vi "JKISM++ Example - Caller is JKISM.vi"() -> ()   [LabVIEW 2014]
uses:
  user.lib/_NEVSTOP/JKI State Machine++/_Polymophic/Build Asynchronous Message with Arguments.vi
  user.lib/_NEVSTOP/JKI State Machine++/_Polymophic/Build No-Reply Asynchronous Message with Arguments.vi
  user.lib/_NEVSTOP/JKI State Machine++/_Polymophic/Build Register Status Message.vi
  user.lib/_NEVSTOP/JKI State Machine++/_Polymophic/Build Unregister Status Message.vi
  user.lib/_NEVSTOP/JKI State Machine++/_Polymophic/Build Synchronous Message with Arguments.vi
  user.lib/_NEVSTOP/JKI State Machine++/_Support/JKISMQ/_Obtain JKISMQ.vi
  user.lib/_NEVSTOP/JKI State Machine++/_Support/FGV-BroadcastRegistry/Cache-Broadcast Registry Search Result.vi
  user.lib/_NEVSTOP/JKI State Machine++/AdvanceAPI/JKISM++ Register Status Change.vi
  user.lib/_NEVSTOP/JKI State Machine++/AdvanceAPI/JKISM++ Unregister Status Change.vi
  user.lib/_NEVSTOP/JKI State Machine++/_Support/JKISMQ/_Create Resp Queue.vi
  user.lib/_NEVSTOP/JKI State Machine++/_Support/JKISMQ/_Unlock JKISMQ.vi
  user.lib/_NEVSTOP/JKI State Machine++/_Support/JKISMQ/_Lock State JKISMQ.vi
  user.lib/_NEVSTOP/JKI State Machine++/_Support/JKISMQ/_Release JKISMQ.vi
  user.lib/_NEVSTOP/JKI State Machine++/AdvanceAPI/JKISM++ Make String Arguments Safe.vi
  user.lib/_NEVSTOP/JKI State Machine++/_Support/Message/Parse State with Arguments String.vi
  user.lib/_NEVSTOP/JKI State Machine++/Utility/Trim Both Whitespace.vi
  user.lib/_NEVSTOP/JKI State Machine++/_Support/JKISMQ/_Input Name to JKISM Mode.vi
  user.lib/_NEVSTOP/JKI State Machine++/Utility/uuid.vi
  user.lib/_NEVSTOP/JKI State Machine++/_Support/KeyWords.vi
  user.lib/_NEVSTOP/JKI State Machine++/_Support/JKISMQ/_JKISMQFGV.vi
  user.lib/_NEVSTOP/JKI State Machine++/_Support/GlobalEvent/FGV-GlobalEventRef.vi
  user.lib/_NEVSTOP/JKI State Machine++/_Support/JKISMQ/_Dequeue JKISMQ.vi
  user.lib/_NEVSTOP/JKI State Machine++/_Support/JKISMQ/_Enqueue JKISMQ.vi
  user.lib/_NEVSTOP/JKI State Machine++/_Support/GlobalEvent/FGV-StatusChangeEventRef.vi
  user.lib/_NEVSTOP/JKI State Machine++/_Support/FGV-BroadcastRegistry/global-Broadcast Cache Change Flag.vi
  user.lib/_NEVSTOP/JKI State Machine++/_Support/FGV-BroadcastRegistry/FGV-BroadcastRegistry.vi
  user.lib/_NEVSTOP/JKI State Machine++/JKI State Machine++.lvlib
panel:
  in  "UI: Front Panel State >> Close":bool
  in  "UI: Front Panel State >> Open":bool
  in  "Level":dbl min=0.0 max=1.0 step=0.1
  in  "Target Module":string(combo)="SubModule0"
  in  "API: Stop":bool
  in  "API: Start":bool
  in  "Unregister All Status Change":bool
  in  "Register All Status Change":bool
  in  "API: Get Level(Async)":bool
  out "State History of Main":string
  # "1. The purpose of this example is to demonstrate how to invoke the JKISM module in the JKISM++ framework program. In this scenario, inter-module communication solely relies on message string queue operations. You can generate a Message string using the \"Build Message with Arguments++.vi\" function. Alternatively, if you are familiar with the rules, you can directly utilize message description strings. \n\nThis example synchronously calls two instances of \"JKISM-Reuse Module.vi\", providing dynamic subscription to status and manipulation of the underlying Module through the API."
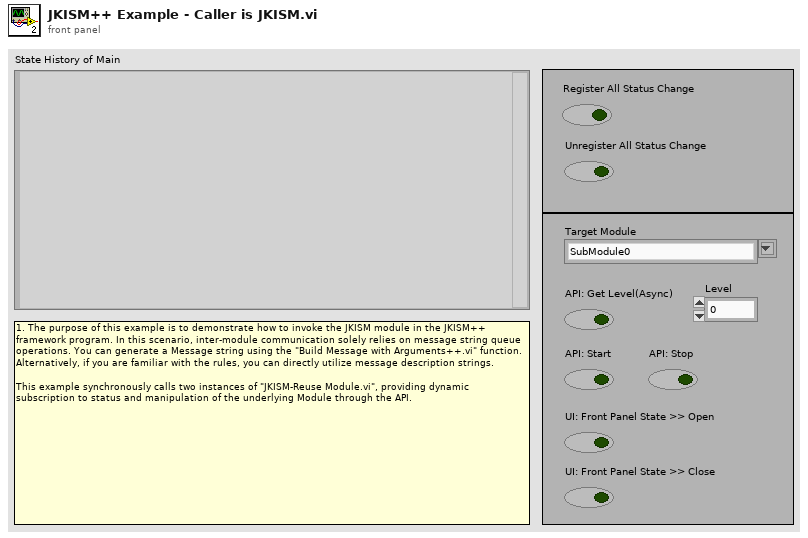
[diagram p1: front panel]
types:
  T1 = enum32{"Invalid", "Standard", "Closed", "Hidden", "Minimized", "Maximized"}
  T2 = enum32{"invalid app kind", "Development System", "Run Time System", "Student Edition", "Embedded LabVIEW", "Evaluation", "Custom"}
  T3 = cluster{"Core":cluster{"Current VI Reference":refnum<vi>, "Close Panel on Exit?":bool}, "Your Boolean data":bool, "Your string data":string, "Active Module":string}
  T4 = cluster{"Current VI Reference":refnum<vi>, "Close Panel on Exit?":bool}
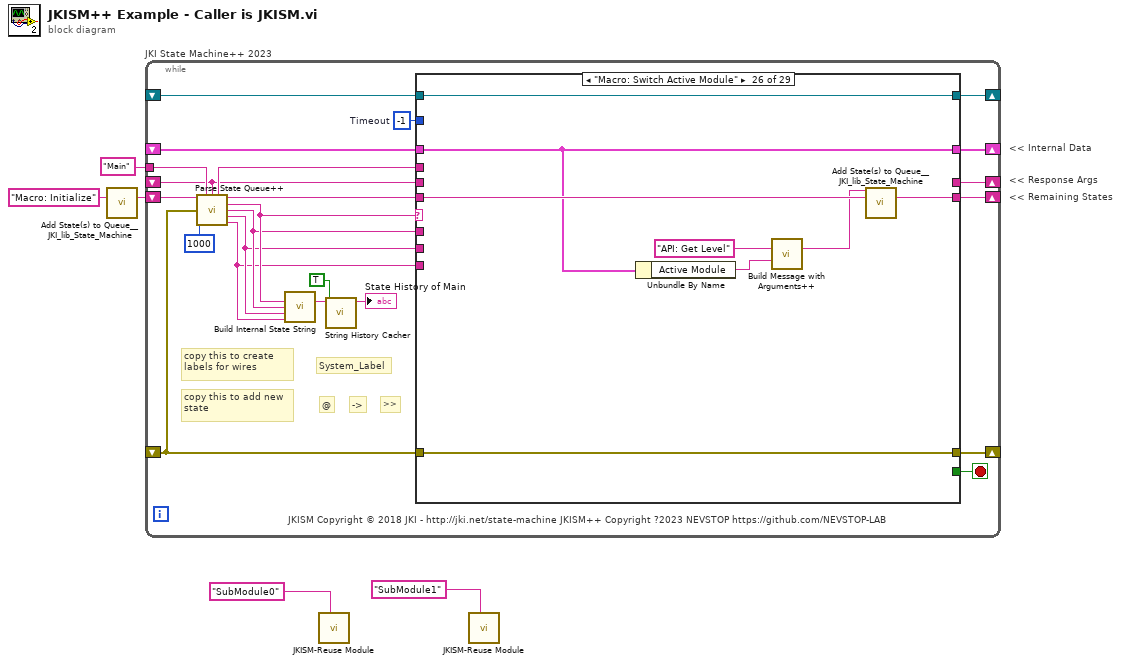
[diagram p0: block diagram]
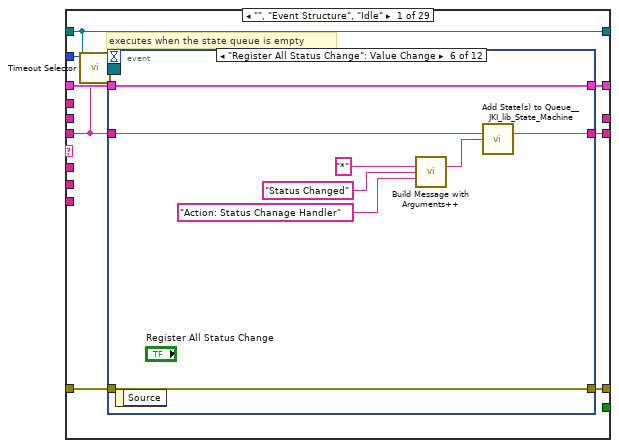
[diagram p2: hidden frame]
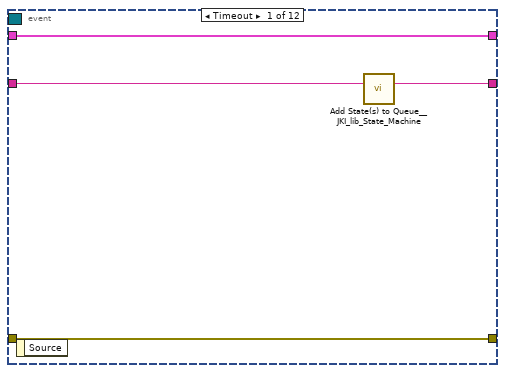
[diagram p3: hidden frame]
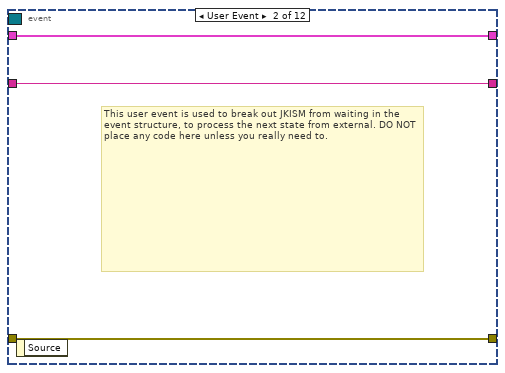
[diagram p4: hidden frame]
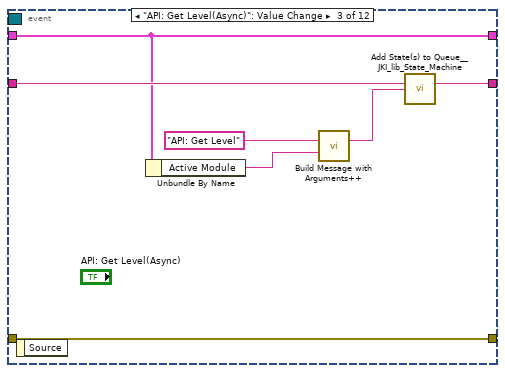
[diagram p5: hidden frame]
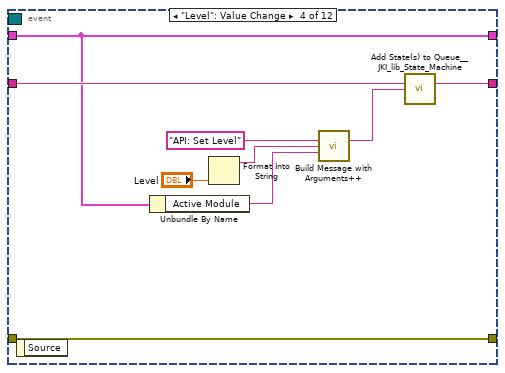
[diagram p6: hidden frame]
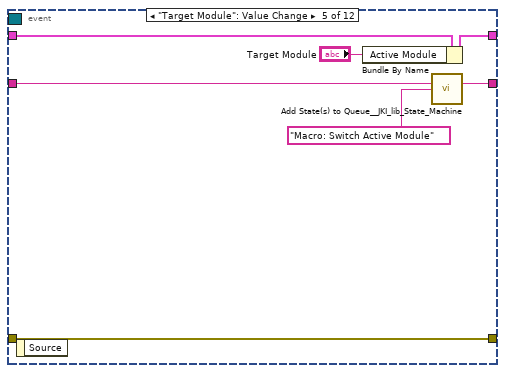
[diagram p7: hidden frame]
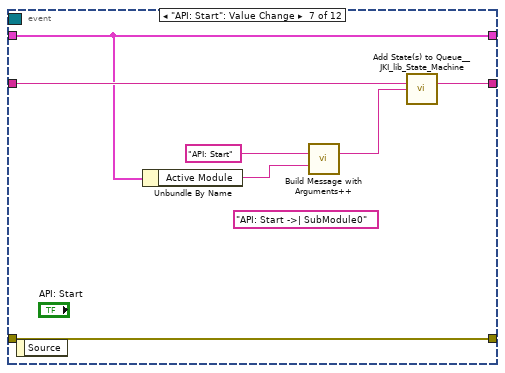
[diagram p8: hidden frame]
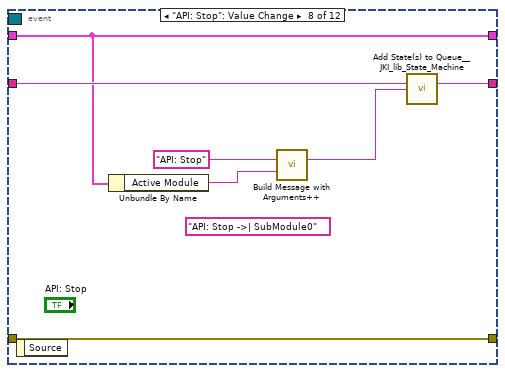
[diagram p9: hidden frame]
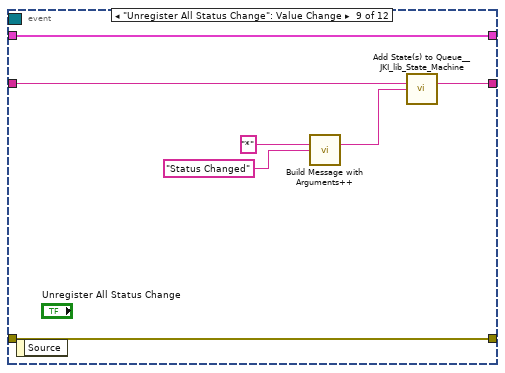
[diagram p10: hidden frame]
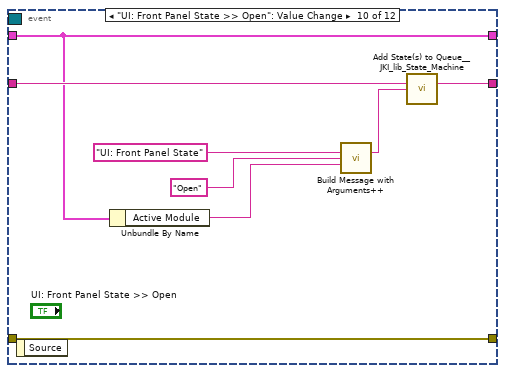
[diagram p11: hidden frame]
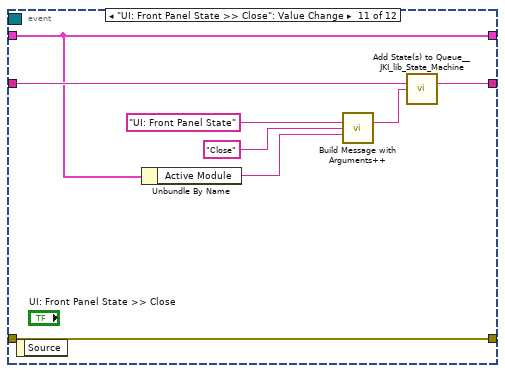
[diagram p12: hidden frame]
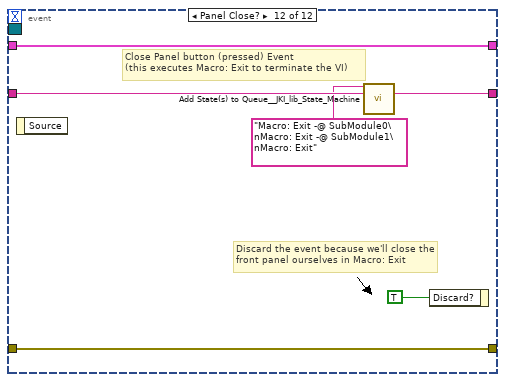
[diagram p13: hidden frame]
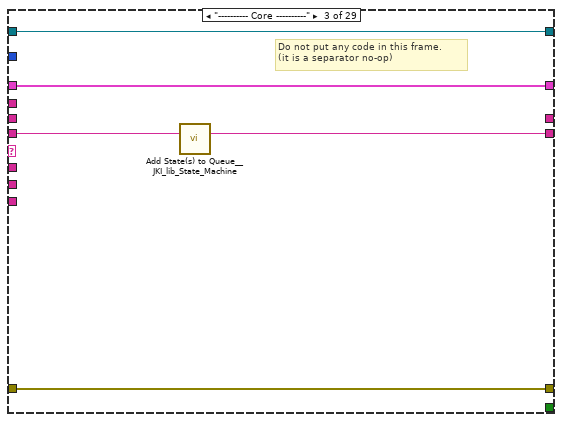
[diagram p15: hidden frame]
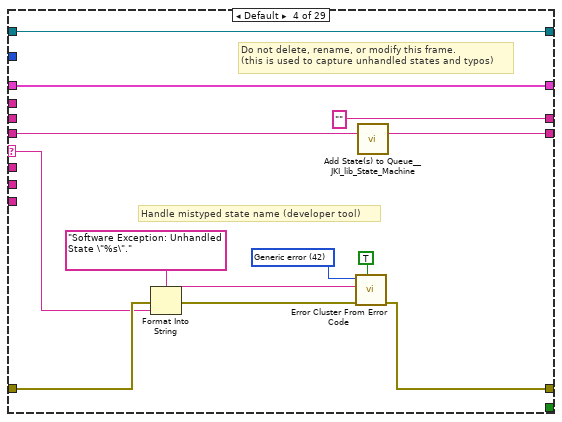
[diagram p16: hidden frame]
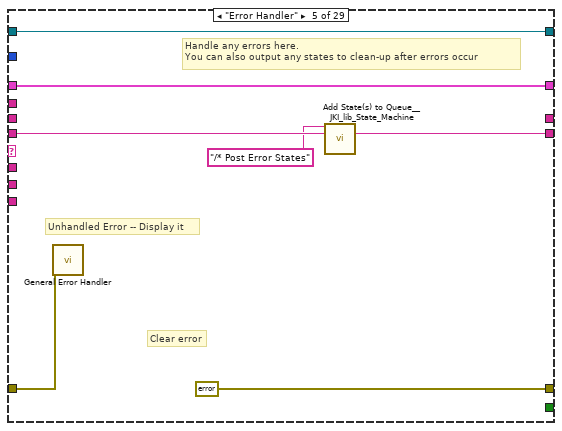
[diagram p17: hidden frame]
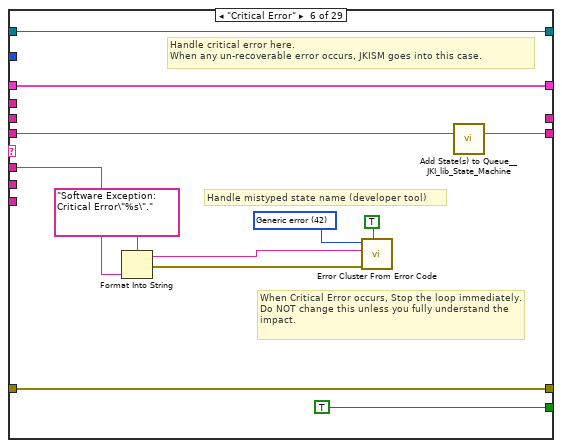
[diagram p18: hidden frame]
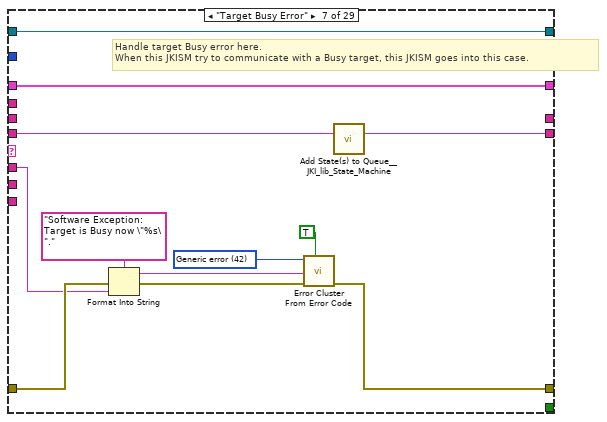
[diagram p19: hidden frame]
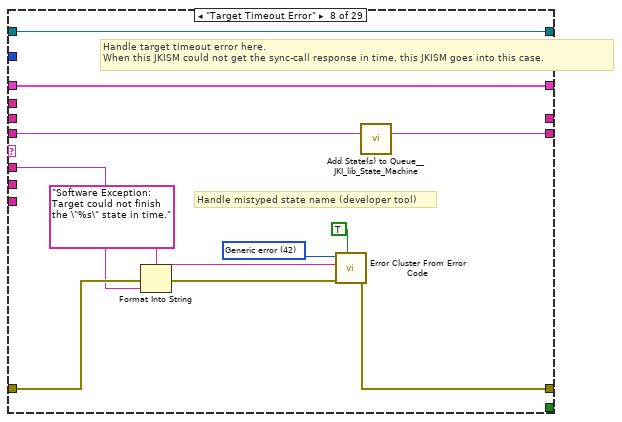
[diagram p20: hidden frame]
diagram:
  # "<< Internal Data"
  # "<< Response Args"
  # "<< Remaining States"
  n1 = call <vilib>:"Add State(s) to Queue__JKI_lib_State_Machine.vi"("State(s) in (\"\")"="Macro: Initialize") -> ("States Out"=w5:string)  [unwired: 14 in]
  n2 = while "JKI State Machine++ 2023" {
    shift-right: [w23] -> _
    shift-left: _ -> [w22]
    shift-right: [w26] -> _
    shift-left: _ -> [w20]
    shift-right: [w25] -> _
    shift-left: w5 -> [w27]
    tunnel: "Main" ("Name(\"\" to use uuid)") -> [w15]
    shift-right: [w18] -> _
    shift-left: _ -> [w7]
    shift-right: [w17] -> _
    shift-left: _ -> [w16]
    stop <- w24 stop-if-true
    w21 = -1  # Timeout
    # "JKISM Copyright © 2018 JKI - http://jki.net/state-machine JKISM++ Copyright ?2023 NEVSTOP https://github.com/NEVSTOP-LAB"
    # "copy this to add new state"
    # ">>"
    # "->"
    # "@"
    # "copy this to create labels for wires"
    # "System_Label"
    n3 = call "Parse State Queue++.vi"("State Queue"=w27, "Name(\"\" to use uuid)"=w15, "Response Arguments"=w7, "Error In (no error)"=w20, "Response Timeout(5000ms)"=1000 ("Response Timeout(1000ms)")) -> ("Name Used"=w8:string, "Remaining States"=w28:string, "Current State"=w12:string, "Arguments"=w11:string, "Argument - State"=w10:string, "From Who"=w9:string)  [unwired: 5 in]
    n4 = call "Build Internal State String.vi"("State"=w12, "Arguments (\"\")"=w11, "Arg-State (\"\")"=w10, "Source (\"\")"=w9) -> ("State with Arguments"=w13:string)  [unwired: 11 in]
    n5 = call "String History Cacher.vi"("Include Timestamp(T)"=TRUE ("Include Timestamp(F)"), "String"=w13) -> ("String Cache"=→"State History of Main":string)  [unwired: 9 in]
    n6 = case shown="\"Macro: Switch Active Module\"" w12 {
      selector: w12 -> [_ _ _ w130 _ _ _ _ _ _ _ _ _ _ _ _ _ _ _ _ _ _ _ _ _ _ _ _ _]
      tunnel: w28 -> [w29 w121 w127 w134 w147 w157 w160 w177 w189 w200 w206 w221 w227 w232 w241 w248 w253 w259 w263 w269 w275 w282 w294 w364 w370 w375 w389 w392 w396]
      tunnel: w11 -> [_ _ _ _ _ w150 w162 w173 w185 w196 _ _ _ _ _ _ _ _ _ _ _ w277 w288 _ _ _ _ _ _]
      tunnel: w22 -> [w36 w120 w124 w132 w144 w158 w164 w175 w187 w199 w205 w214 w225 w229 _ w243 w250 w258 w262 w266 w271 w280 w290 w361 w367 w373 w386 w391 w395]
      tunnel: [w35 w122 w125 w136 errorcluster {"status"=FALSE, "code"=0, "source"=""} ("error out") w159 w167 w179 w191 w201 w207 w218 w224 w230 w238 w244 w251 w254 w261 w267 w273 w278 w291 w362 w368 w378 w387 w393 w397] -> w26
      tunnel: w20 -> [w34 w122 w125 w135 w143 w159 w166 w178 w190 w201 w207 w218 w224 w230 w238 w245 w251 _ w264 w267 w273 w279 w292 w362 w368 w378 w387 w393 w397]
      tunnel: [w37 w121 w126 w133 w146 w156 w165 w176 w188 w200 w206 w220 w226 w231 w240 w247 w252 w259 w263 w268 w274 w281 w293 w363 w369 w376 w388 w392 w396] -> w25
      tunnel: [_ _ _ _ _ TRUE _ _ _ _ _ _ TRUE _ _ _ _ _ _ _ _ _ _ _ _ _ _ _ _] -> w24
      tunnel: [w33 w120 w124 w132 w144 w158 w164 w175 w187 w199 w205 w219 w225 w229 w239 w243 w250 w258 w262 w266 w271 w280 w290 w361 w367 w373 w386 w391 w395] -> w23
      tunnel: w21 -> [w32 _ _ _ _ _ _ _ _ _ _ _ _ _ _ _ _ _ _ _ _ _ _ _ _ _ _ _ _]
      tunnel: w9 -> [_ _ _ _ _ _ _ _ _ _ _ _ _ _ _ _ _ _ _ _ _ _ _ _ _ _ _ _ _]
      tunnel: w10 -> [_ _ _ _ _ _ _ _ _ w197 _ _ _ _ _ _ _ _ _ _ _ _ _ _ _ _ _ _ _]
      tunnel: [_ _ _ "" _ _ _ _ _ _ _ _ _ _ _ _ _ _ _ _ _ _ _ _ _ _ _ _ _] -> w18
      tunnel: [w31 w119 w123 w128 w141 w148 w161 w172 w184 w198 w204 w208 w222 w228 w234 w242 w249 w257 w260 w265 w272 w276 w287 w360 w365 w377 w379 w390 w394] -> w17
      tunnel: w16 -> [w31 w119 w123 w128 w141 w148 w161 w172 w184 w198 w204 w208 w222 w228 w234 w242 w249 _ w260 w265 w272 w276 w287 w360 w365 w377 w379 w390 w394]
      tunnel: w8 -> [_ _ _ _ _ _ _ _ _ _ _ _ _ _ _ _ _ w256 _ _ _ _ _ _ _ _ _ _ _]
      tunnel: w7 -> [_ _ _ _ _ _ _ _ _ _ _ _ _ _ _ _ _ _ _ _ _ _ _ _ _ _ _ _ _]
      frame "", "Event Structure", "Idle" {
        # "executes when the state queue is empty"
        n7 = call "Timeout Selector.vi"("Remaining States"=w29, "Timeout Expected"=w32) -> ("Timeout"=w30:i32)  [unwired: 5 in]
        n8 = event shown="[5] \"Register All Status Change\": Value Change" {
          selector: w31 -> [_ _ _ _ _ _ _ _ _ _ _ _]
          dyn-events: _ -> [_ _ _ _ _ _ _ _ _ _ _ _]
          timeout: w30 -> [_ _ _ _ _ _ _ _ _ _ _ _]
          tunnel: w29 -> [w41 w43 w50 w59 w64 w73 w81 w88 w94 w103 w111 w118]
          tunnel: [w40 w43 w49 w58 w65 w72 w80 w87 w93 w102 w110 w117] -> w37
          tunnel: w36 -> [w38 w44 w46 w53 w66 w74 w77 w84 w95 w101 w108 w115]
          tunnel: [w39 w42 w51 w60 w67 w75 w82 w89 w96 w104 w112 w116] -> w35
          tunnel: w34 -> [w39 w42 w51 w60 w67 w75 w82 w89 w96 w104 w112 w116]
          tunnel: [w38 w44 w46 w53 w62 w74 w77 w84 w95 w101 w108 w115] -> w33
          event Timeout {
            n9 = event-data() -> ()  [unwired: 1 in, 1 out]
            n10 = call <vilib>:"Add State(s) to Queue__JKI_lib_State_Machine.vi"("State(s) in (\"\")"=w41) -> ("States Out"=w40:string)  [unwired: 14 in]
          }
          event User Event {
            # "This user event is used to break out JKISM from waiting in the event structure, to process the next state from external. DO NOT place any code here unless you really need to."
            n11 = event-data() -> ()  [unwired: 1 in, 1 out]
          }
          event "API: Get Level(Async)": Value Change {
            n12 = event-data() -> ()  [unwired: 1 in, 1 out]
            n13 = Unbundle By Name(w46) -> ("Active Module"=w45:string)
            n14 = call-poly "Build Message with Arguments++.vi"("State with Arguments"="API: Get Level" ("State(s) in Front (\"\")"), "Target Module (\"\")"=w45) -> ("State with Arguments"=w47:string)  [unwired: 13 in]
            n15 = call <vilib>:"Add State(s) to Queue__JKI_lib_State_Machine.vi"("State(s) in (\"\")"=w50, "State(s) at Back (\"\")"=w47) -> ("States Out"=w49:string)  [unwired: 13 in]
          }
          event "Level": Value Change {
            n16 = event-data() -> ()  [unwired: 1 in, 1 out]
            n17 = Unbundle By Name(w53) -> ("Active Module"=w52:string)
            n18 = Format Into String("Level") -> (resulting string=w54:string)  [unwired: 3 in, 1 out]
            n19 = call-poly "Build Message with Arguments++.vi"("State with Arguments"="API: Set Level" ("State(s) in Front (\"\")"), "Arguments (\"\")"=w54, "Target Module (\"\")"=w52) -> ("State with Arguments"=w56:string)  [unwired: 12 in]
            n20 = call <vilib>:"Add State(s) to Queue__JKI_lib_State_Machine.vi"("State(s) in (\"\")"=w59, "State(s) at Back (\"\")"=w56) -> ("States Out"=w58:string)  [unwired: 13 in]
          }
          event "Target Module": Value Change {
            n21 = event-data() -> ()  [unwired: 1 in, 1 out]
            n22 = Bundle By Name(cluster=w66, "Active Module"="Target Module") -> (w62:T3)
            n23 = call <vilib>:"Add State(s) to Queue__JKI_lib_State_Machine.vi"("State(s) in (\"\")"=w64, "State(s) at Back (\"\")"="Macro: Switch Active Module" ("State(s) at Back (\"\")")) -> ("States Out"=w65:string)  [unwired: 13 in]
          }
          event "Register All Status Change": Value Change {
            n24 = event-data() -> ()  [unwired: 1 in, 1 out]
            n25 = call-poly "Build Message with Arguments++.vi"("Source JKISM Name (* as Default)"="*", "Status"="Status Changed", "Response Message (if \"\", same as Source Message)"="Action: Status Chanage Handler" ("Status")) -> ("State with Arguments"=w68:string)  [unwired: 12 in]
            n26 = call <vilib>:"Add State(s) to Queue__JKI_lib_State_Machine.vi"("State(s) in (\"\")"=w73, "State(s) at Back (\"\")"=w68) -> ("States Out"=w72:string)  [unwired: 13 in]
          }
          event "API: Start": Value Change {
            (unwired) "API: Start ->| SubModule0" ("State(s) in Front (\"\")")
            n27 = event-data() -> ()  [unwired: 1 in, 1 out]
            n28 = Unbundle By Name(w77) -> ("Active Module"=w76:string)
            n29 = call-poly "Build Message with Arguments++.vi"("State with Arguments"="API: Start" ("State(s) in Front (\"\")"), "Target Module (\"\")"=w76) -> ("State with Arguments"=w78:string)  [unwired: 13 in]
            n30 = call <vilib>:"Add State(s) to Queue__JKI_lib_State_Machine.vi"("State(s) in (\"\")"=w81, "State(s) at Back (\"\")"=w78) -> ("States Out"=w80:string)  [unwired: 13 in]
          }
          event "API: Stop": Value Change {
            (unwired) "API: Stop ->| SubModule0" ("State(s) in Front (\"\")")
            n31 = event-data() -> ()  [unwired: 1 in, 1 out]
            n32 = Unbundle By Name(w84) -> ("Active Module"=w83:string)
            n33 = call-poly "Build Message with Arguments++.vi"("State with Arguments"="API: Stop" ("State(s) in Front (\"\")"), "Target Module (\"\")"=w83) -> ("State with Arguments"=w85:string)  [unwired: 13 in]
            n34 = call <vilib>:"Add State(s) to Queue__JKI_lib_State_Machine.vi"("State(s) in (\"\")"=w88, "State(s) at Back (\"\")"=w85) -> ("States Out"=w87:string)  [unwired: 13 in]
          }
          event "Unregister All Status Change": Value Change {
            n35 = event-data() -> ()  [unwired: 1 in, 1 out]
            n36 = call-poly "Build Message with Arguments++.vi"("Source JKISM Name (* as Default)"="*", "Status"="Status Changed") -> ("State with Arguments"=w90:string)  [unwired: 13 in]
            n37 = call <vilib>:"Add State(s) to Queue__JKI_lib_State_Machine.vi"("State(s) in (\"\")"=w94, "State(s) at Back (\"\")"=w90) -> ("States Out"=w93:string)  [unwired: 13 in]
          }
          event "UI: Front Panel State >> Open": Value Change {
            n38 = event-data() -> ()  [unwired: 1 in, 1 out]
            n39 = Unbundle By Name(w101) -> ("Active Module"=w100:string)
            n40 = call-poly "Build Message with Arguments++.vi"("State with Arguments"="UI: Front Panel State" ("JKISM Name"), "Arguments (\"\")"="Open" ("JKISM Name"), "Target Module (\"\")"=w100) -> ("State with Arguments"=w99:string)  [unwired: 12 in]
            n41 = call <vilib>:"Add State(s) to Queue__JKI_lib_State_Machine.vi"("State(s) in (\"\")"=w103, "State(s) at Back (\"\")"=w99) -> ("States Out"=w102:string)  [unwired: 13 in]
          }
          event "UI: Front Panel State >> Close": Value Change {
            n42 = event-data() -> ()  [unwired: 1 in, 1 out]
            n43 = Unbundle By Name(w108) -> ("Active Module"=w107:string)
            n44 = call-poly "Build Message with Arguments++.vi"("State with Arguments"="UI: Front Panel State" ("JKISM Name"), "Arguments (\"\")"="Close" ("JKISM Name"), "Target Module (\"\")"=w107) -> ("State with Arguments"=w106:string)  [unwired: 12 in]
            n45 = call <vilib>:"Add State(s) to Queue__JKI_lib_State_Machine.vi"("State(s) in (\"\")"=w111, "State(s) at Back (\"\")"=w106) -> ("States Out"=w110:string)  [unwired: 13 in]
          }
          event Panel Close? {
            # "Discard the event because we'll close the front panel ourselves in Macro: Exit"
            # "Close Panel button (pressed) Event\n(this executes Macro: Exit to terminate the VI)"
            n46 = event-data() -> ()  [unwired: 1 in, 1 out]
            n47 = call <vilib>:"Add State(s) to Queue__JKI_lib_State_Machine.vi"("State(s) in Front (\"\")"="Macro: Exit -@ SubModule0\nMacro: Exit -@ SubModule1\nMacro: Exit", "State(s) in (\"\")"=w118) -> ("States Out"=w117:string)  [unwired: 13 in]
            n48 = event-data("Discard?"=TRUE) -> ()  [unwired: 1 in, 1 out]
          }
        }
      }
      frame "JKISM++ Documentation" {
        # "Commenting:\nTo add a comment use \"//\" or \"#\" and all text to the right will be ignored\nCommenting Example:\nUI: Initialize // This initializes the UI\n# This whole line is a comment\n// Another comment line"
        # "State Syntax:\nStateCategory: State >> Argument @ JKISMName\nStateCategory: State >> Argument -> JKISMName\n\nLine Terminator: Line feed"
        # "JKISM++ Documentation"
      }
      frame "---------- Core ----------" {
        # "Do not put any code in this frame.\n(it is a separator no-op)"
        n49 = call <vilib>:"Add State(s) to Queue__JKI_lib_State_Machine.vi"("State(s) in (\"\")"=w127) -> ("States Out"=w126:string)  [unwired: 14 in]
      }
      frame Default {
        w139 = 42 items=["No error", "Argument error", "Memory is full", "Out of zone", "End of file", "File already open", "Generic file I/O error", "File not found", "File permission error", "Disk is full", "Duplicate path", "Too many files open", "System feature not enabled", "Resource file not found", "Cannot add resource", "Resource not found", "Image not found", "Image memory error", "Pen does not exist", "Config type invalid", "Config token not found", "Config parse error", "Config memory error", "Bad external code format", "Bad external code offset", "External code not present", "Null window", "Destroy window error", "Null menu", "Print aborted", "Bad print record", "Print driver error", "Windows error during printing", "Memory error during printing", "Print dialog error", "Generic print error", "Invalid device refnum", "Device not found", "Device parameter error", "Device unit error", "Cannot open device", "Device call aborted", "Generic error", "Cancelled by user", "Object ID too low", "Object ID too high", "Object not in heap", "Unknown heap", "Unknown object (invalid DefProc)", "Unknown object (DefProc not in table)", "Message out of range", "Invalid (null) method", "Unknown message", "Manager call not supported", "Bad address", "Network operation in progress", "Network operation timed out", "Connection is busy", "Network attribute not supported", "Network error", "Address in use", "System out of memory", "Connection aborted", "Connection refused", "Not connected", "Already connected", "Connection closed", "Initialization error (interapplication manager)", "Bad occurrence", "Wait on unbound occurrence handler", "Occurrence queue overflow", "Datalog type conflict", "Unused", "Unrecognized type (interapplication manager)", "Memory corrupt", "Failed to make temporary DLL", "Old CIN version", "Drag socket not found", "Failed to load drop-object", "Failed to register OLE object", "Failed to release OLE object", "Format specifier type mismatch", "Unknown format specifier", "Too few format specifiers", "Too many format specifiers", "Scan failed", "Newer CIN version", "Error converting to variant", "Runtime menu error", "Password tampered", "Variant attribute not found", "Incompatible variant data type", "Event data is not available", "Event Store is not present", "Occurrence is not found", "Event Queue is not created", "Event info is not available", "Refnum passed is NULL", "Error retrieving Class GUID", "Error retrieving CoClass GUID", "Error retrieving TypeLib GUID.", "Bad built application magic bytes.", "Specific driver is different from the specific driver associated with the Logical Name.", "There is no session opened to the class driver.", "Max Error", "MAX - Error with config objects", "MAX - Error loading configuration", "MAX - Group not supported"]
        # "Do not delete, rename, or modify this frame.\n(this is used to capture unhandled states and typos)"
        # "Handle mistyped state name (developer tool)"
        n50 = Format Into String(format string="Software Exception: Unhandled State \"%s\"." ("message"), error in=w135, w130) -> (resulting string=w138:string, error out=w137:errorcluster)  [unwired: 1 in]
        n51 = call <vilib>:"Error Cluster From Error Code.vi"("show call chain? (False)"=TRUE, "error in (no error)"=w137, "error message (\"\")"=w138, "error code (0)"=w139) -> ("error out"=w136:errorcluster)  [unwired: 5 in]
        n52 = call <vilib>:"Add State(s) to Queue__JKI_lib_State_Machine.vi"("State(s) in (\"\")"=w134) -> ("States Out"=w133:string)  [unwired: 14 in]
      }
      frame "Error Handler" {
        # "Unhandled Error -- Display it"
        # "Handle any errors here.\nYou can also output any states to clean-up after errors occur"
        # "Clear error"
        n53 = call <vilib>:"General Error Handler.vi"("error in (no error)"=w143) -> ()  [unwired: 10 in, 5 out]
        n54 = call <vilib>:"Add State(s) to Queue__JKI_lib_State_Machine.vi"("State(s) in Front (\"\")"="/* Post Error States", "State(s) in (\"\")"=w147) -> ("States Out"=w146:string)  [unwired: 13 in]
      }
      frame "Critical Error" {
        w154 = 42 items=["No error", "Argument error", "Memory is full", "Out of zone", "End of file", "File already open", "Generic file I/O error", "File not found", "File permission error", "Disk is full", "Duplicate path", "Too many files open", "System feature not enabled", "Resource file not found", "Cannot add resource", "Resource not found", "Image not found", "Image memory error", "Pen does not exist", "Config type invalid", "Config token not found", "Config parse error", "Config memory error", "Bad external code format", "Bad external code offset", "External code not present", "Null window", "Destroy window error", "Null menu", "Print aborted", "Bad print record", "Print driver error", "Windows error during printing", "Memory error during printing", "Print dialog error", "Generic print error", "Invalid device refnum", "Device not found", "Device parameter error", "Device unit error", "Cannot open device", "Device call aborted", "Generic error", "Cancelled by user", "Object ID too low", "Object ID too high", "Object not in heap", "Unknown heap", "Unknown object (invalid DefProc)", "Unknown object (DefProc not in table)", "Message out of range", "Invalid (null) method", "Unknown message", "Manager call not supported", "Bad address", "Network operation in progress", "Network operation timed out", "Connection is busy", "Network attribute not supported", "Network error", "Address in use", "System out of memory", "Connection aborted", "Connection refused", "Not connected", "Already connected", "Connection closed", "Initialization error (interapplication manager)", "Bad occurrence", "Wait on unbound occurrence handler", "Occurrence queue overflow", "Datalog type conflict", "Unused", "Unrecognized type (interapplication manager)", "Memory corrupt", "Failed to make temporary DLL", "Old CIN version", "Drag socket not found", "Failed to load drop-object", "Failed to register OLE object", "Failed to release OLE object", "Format specifier type mismatch", "Unknown format specifier", "Too few format specifiers", "Too many format specifiers", "Scan failed", "Newer CIN version", "Error converting to variant", "Runtime menu error", "Password tampered", "Variant attribute not found", "Incompatible variant data type", "Event data is not available", "Event Store is not present", "Occurrence is not found", "Event Queue is not created", "Event info is not available", "Refnum passed is NULL", "Error retrieving Class GUID", "Error retrieving CoClass GUID", "Error retrieving TypeLib GUID.", "Bad built application magic bytes.", "Specific driver is different from the specific driver associated with the Logical Name.", "There is no session opened to the class driver.", "Max Error", "MAX - Error with config objects", "MAX - Error loading configuration", "MAX - Group not supported"]
        # "Handle critical error here.\nWhen any un-recoverable error occurs, JKISM goes into this case."
        # "When Critical Error occurs, Stop the loop immediately. Do NOT change this unless you fully understand the impact."
        # "Handle mistyped state name (developer tool)"
        n55 = Format Into String(format string="Software Exception: Critical Error\"%s\"." ("message"), w150) -> (resulting string=w153:string, error out=w152:errorcluster)  [unwired: 2 in]
        n56 = call <vilib>:"Error Cluster From Error Code.vi"("show call chain? (False)"=TRUE, "error in (no error)"=w152, "error message (\"\")"=w153, "error code (0)"=w154) -> ()  [unwired: 5 in, 1 out]
        n57 = call <vilib>:"Add State(s) to Queue__JKI_lib_State_Machine.vi"("State(s) in (\"\")"=w157) -> ("States Out"=w156:string)  [unwired: 14 in]
      }
      frame "Target Busy Error" {
        w170 = 42 items=["No error", "Argument error", "Memory is full", "Out of zone", "End of file", "File already open", "Generic file I/O error", "File not found", "File permission error", "Disk is full", "Duplicate path", "Too many files open", "System feature not enabled", "Resource file not found", "Cannot add resource", "Resource not found", "Image not found", "Image memory error", "Pen does not exist", "Config type invalid", "Config token not found", "Config parse error", "Config memory error", "Bad external code format", "Bad external code offset", "External code not present", "Null window", "Destroy window error", "Null menu", "Print aborted", "Bad print record", "Print driver error", "Windows error during printing", "Memory error during printing", "Print dialog error", "Generic print error", "Invalid device refnum", "Device not found", "Device parameter error", "Device unit error", "Cannot open device", "Device call aborted", "Generic error", "Cancelled by user", "Object ID too low", "Object ID too high", "Object not in heap", "Unknown heap", "Unknown object (invalid DefProc)", "Unknown object (DefProc not in table)", "Message out of range", "Invalid (null) method", "Unknown message", "Manager call not supported", "Bad address", "Network operation in progress", "Network operation timed out", "Connection is busy", "Network attribute not supported", "Network error", "Address in use", "System out of memory", "Connection aborted", "Connection refused", "Not connected", "Already connected", "Connection closed", "Initialization error (interapplication manager)", "Bad occurrence", "Wait on unbound occurrence handler", "Occurrence queue overflow", "Datalog type conflict", "Unused", "Unrecognized type (interapplication manager)", "Memory corrupt", "Failed to make temporary DLL", "Old CIN version", "Drag socket not found", "Failed to load drop-object", "Failed to register OLE object", "Failed to release OLE object", "Format specifier type mismatch", "Unknown format specifier", "Too few format specifiers", "Too many format specifiers", "Scan failed", "Newer CIN version", "Error converting to variant", "Runtime menu error", "Password tampered", "Variant attribute not found", "Incompatible variant data type", "Event data is not available", "Event Store is not present", "Occurrence is not found", "Event Queue is not created", "Event info is not available", "Refnum passed is NULL", "Error retrieving Class GUID", "Error retrieving CoClass GUID", "Error retrieving TypeLib GUID.", "Bad built application magic bytes.", "Specific driver is different from the specific driver associated with the Logical Name.", "There is no session opened to the class driver.", "Max Error", "MAX - Error with config objects", "MAX - Error loading configuration", "MAX - Group not supported"]
        # "Handle target Busy error here.\nWhen this JKISM try to communicate with a Busy target, this JKISM goes into this case."
        n58 = Format Into String(format string="Software Exception: Target is Busy now \"%s\"." ("message"), error in=w166, w162) -> (resulting string=w169:string, error out=w168:errorcluster)  [unwired: 1 in]
        n59 = call <vilib>:"Error Cluster From Error Code.vi"("show call chain? (False)"=TRUE, "error in (no error)"=w168, "error message (\"\")"=w169, "error code (0)"=w170) -> ("error out"=w167:errorcluster)  [unwired: 5 in]
        n60 = call <vilib>:"Add State(s) to Queue__JKI_lib_State_Machine.vi"("State(s) in (\"\")"=w160) -> ("States Out"=w165:string)  [unwired: 14 in]
      }
      frame "Target Timeout Error" {
        w182 = 42 items=["No error", "Argument error", "Memory is full", "Out of zone", "End of file", "File already open", "Generic file I/O error", "File not found", "File permission error", "Disk is full", "Duplicate path", "Too many files open", "System feature not enabled", "Resource file not found", "Cannot add resource", "Resource not found", "Image not found", "Image memory error", "Pen does not exist", "Config type invalid", "Config token not found", "Config parse error", "Config memory error", "Bad external code format", "Bad external code offset", "External code not present", "Null window", "Destroy window error", "Null menu", "Print aborted", "Bad print record", "Print driver error", "Windows error during printing", "Memory error during printing", "Print dialog error", "Generic print error", "Invalid device refnum", "Device not found", "Device parameter error", "Device unit error", "Cannot open device", "Device call aborted", "Generic error", "Cancelled by user", "Object ID too low", "Object ID too high", "Object not in heap", "Unknown heap", "Unknown object (invalid DefProc)", "Unknown object (DefProc not in table)", "Message out of range", "Invalid (null) method", "Unknown message", "Manager call not supported", "Bad address", "Network operation in progress", "Network operation timed out", "Connection is busy", "Network attribute not supported", "Network error", "Address in use", "System out of memory", "Connection aborted", "Connection refused", "Not connected", "Already connected", "Connection closed", "Initialization error (interapplication manager)", "Bad occurrence", "Wait on unbound occurrence handler", "Occurrence queue overflow", "Datalog type conflict", "Unused", "Unrecognized type (interapplication manager)", "Memory corrupt", "Failed to make temporary DLL", "Old CIN version", "Drag socket not found", "Failed to load drop-object", "Failed to register OLE object", "Failed to release OLE object", "Format specifier type mismatch", "Unknown format specifier", "Too few format specifiers", "Too many format specifiers", "Scan failed", "Newer CIN version", "Error converting to variant", "Runtime menu error", "Password tampered", "Variant attribute not found", "Incompatible variant data type", "Event data is not available", "Event Store is not present", "Occurrence is not found", "Event Queue is not created", "Event info is not available", "Refnum passed is NULL", "Error retrieving Class GUID", "Error retrieving CoClass GUID", "Error retrieving TypeLib GUID.", "Bad built application magic bytes.", "Specific driver is different from the specific driver associated with the Logical Name.", "There is no session opened to the class driver.", "Max Error", "MAX - Error with config objects", "MAX - Error loading configuration", "MAX - Group not supported"]
        # "Handle target timeout error here.\nWhen this JKISM could not get the sync-call response in time, this JKISM goes into this case."
        # "Handle mistyped state name (developer tool)"
        n61 = Format Into String(format string="Software Exception: Target could not finish the \"%s\" state in time." ("message"), error in=w178, w173) -> (resulting string=w181:string, error out=w180:errorcluster)  [unwired: 1 in]
        n62 = call <vilib>:"Error Cluster From Error Code.vi"("show call chain? (False)"=TRUE, "error in (no error)"=w180, "error message (\"\")"=w181, "error code (0)"=w182) -> ("error out"=w179:errorcluster)  [unwired: 5 in]
        n63 = call <vilib>:"Add State(s) to Queue__JKI_lib_State_Machine.vi"("State(s) in (\"\")"=w177) -> ("States Out"=w176:string)  [unwired: 14 in]
      }
      frame "Target Error" {
        w194 = 42 items=["No error", "Argument error", "Memory is full", "Out of zone", "End of file", "File already open", "Generic file I/O error", "File not found", "File permission error", "Disk is full", "Duplicate path", "Too many files open", "System feature not enabled", "Resource file not found", "Cannot add resource", "Resource not found", "Image not found", "Image memory error", "Pen does not exist", "Config type invalid", "Config token not found", "Config parse error", "Config memory error", "Bad external code format", "Bad external code offset", "External code not present", "Null window", "Destroy window error", "Null menu", "Print aborted", "Bad print record", "Print driver error", "Windows error during printing", "Memory error during printing", "Print dialog error", "Generic print error", "Invalid device refnum", "Device not found", "Device parameter error", "Device unit error", "Cannot open device", "Device call aborted", "Generic error", "Cancelled by user", "Object ID too low", "Object ID too high", "Object not in heap", "Unknown heap", "Unknown object (invalid DefProc)", "Unknown object (DefProc not in table)", "Message out of range", "Invalid (null) method", "Unknown message", "Manager call not supported", "Bad address", "Network operation in progress", "Network operation timed out", "Connection is busy", "Network attribute not supported", "Network error", "Address in use", "System out of memory", "Connection aborted", "Connection refused", "Not connected", "Already connected", "Connection closed", "Initialization error (interapplication manager)", "Bad occurrence", "Wait on unbound occurrence handler", "Occurrence queue overflow", "Datalog type conflict", "Unused", "Unrecognized type (interapplication manager)", "Memory corrupt", "Failed to make temporary DLL", "Old CIN version", "Drag socket not found", "Failed to load drop-object", "Failed to register OLE object", "Failed to release OLE object", "Format specifier type mismatch", "Unknown format specifier", "Too few format specifiers", "Too many format specifiers", "Scan failed", "Newer CIN version", "Error converting to variant", "Runtime menu error", "Password tampered", "Variant attribute not found", "Incompatible variant data type", "Event data is not available", "Event Store is not present", "Occurrence is not found", "Event Queue is not created", "Event info is not available", "Refnum passed is NULL", "Error retrieving Class GUID", "Error retrieving CoClass GUID", "Error retrieving TypeLib GUID.", "Bad built application magic bytes.", "Specific driver is different from the specific driver associated with the Logical Name.", "There is no session opened to the class driver.", "Max Error", "MAX - Error with config objects", "MAX - Error loading configuration", "MAX - Group not supported"]
        # "Handle target error here.\nWhen this JKISM try to communicate with an un-existed JKISM, this JKISM goes into this case."
        # "Handle mistyped state name (developer tool)"
        n64 = Format Into String(format string="Software Exception: Target \"%s\" does not exists." ("message"), error in=w190, w185) -> (resulting string=w193:string, error out=w192:errorcluster)  [unwired: 1 in]
        n65 = call <vilib>:"Add State(s) to Queue__JKI_lib_State_Machine.vi"("State(s) in (\"\")"=w189) -> ("States Out"=w188:string)  [unwired: 14 in]
        n66 = call <vilib>:"Error Cluster From Error Code.vi"("show call chain? (False)"=TRUE, "error in (no error)"=w192, "error message (\"\")"=w193, "error code (0)"=w194) -> ("error out"=w191:errorcluster)  [unwired: 5 in]
      }
      frame "Async Response", "Response" {
        # "Handle Async-call Response (\"Async Response\" for ->)"
        # "Handle Sync-call Response (\"Response\" for @)"
        n67 = case shown="\"API: Get Level\"" w197 {
          tunnel: w196 -> [_ w203]
          frame "False", Default {
          }
          frame "API: Get Level" {
            n68 = Fract/Exp String To Number(string=w203) -> (number=w202:dbl)  [unwired: 3 in, 1 out]
            n69 = local write "Level"(w202) -> ()
          }
        }
      }
      frame "Async Message Posted" {
        # "Handle post action for async message (->)."
        # "After Async Message is posted (->), JKISM+ goes to this state for post-action. You can use Argument - State to tell which Async Message is called."
      }
      frame "Initialize Core Data" {
        # "Do not delete, rename, or modify this frame.\n(this is used to determine panel behavior on exit)"
        # "originally closed?"
        # "exe?"
        # "If panel starts closed or is an EXE, then close it when we exit"
        n70 = property class="VI"() -> ("FP.State"=w211:T1)  [unwired: 2 in, 2 out]
        n71 = property class="App"() -> ("App.Kind"=w217:T2)  [unwired: 2 in, 2 out]
        n72 = control-ref of="Current VI Reference"() -> (w212:refnum<vi>)
        n73 = Equal?(x=w211, y=T1."Closed" ("Front Panel Window:State")) -> (x = y?=w209:bool)
        n74 = Equal?(x=w217, y=T2."Run Time System" ("Application:Kind")) -> (x = y?=w215:bool)
        n75 = Or(x=w209, y=w215) -> (x .or. y?=w213:bool)
        n76 = Bundle By Name(cluster=w214, "Core.Current VI Reference"=w212, "Core.Close Panel on Exit?"=w213) -> (w219:T3)
        n77 = call <vilib>:"Add State(s) to Queue__JKI_lib_State_Machine.vi"("State(s) in (\"\")"=w221) -> ("States Out"=w220:string)  [unwired: 14 in]
      }
      frame "Exit" {
        # "Do not put any code in this frame.\n(No errors that occur here will be handled.)"
        n78 = call <vilib>:"Add State(s) to Queue__JKI_lib_State_Machine.vi"("State(s) in (\"\")"=w227) -> ("States Out"=w226:string)  [unwired: 14 in]
      }
      frame "---------- Data ----------" {
        # "Do not put any code in this frame.\n(It is a separator no-op. You can make a copy of this frame to create a new Data frame)"
        n79 = call <vilib>:"Add State(s) to Queue__JKI_lib_State_Machine.vi"("State(s) in (\"\")"=w232) -> ("States Out"=w231:string)  [unwired: 14 in]
      }
      frame "Data: Initialize" {
        w233 = "SubModule0"  # Active Module
        w235 = T4 {"Current VI Reference"=refnum, "Close Panel on Exit?"=FALSE}  # Core
        w237 = TRUE  # Your Boolean data
        w236 = ""  # Your string data
        # "do not delete - used by framework"
        # "Initialize the shift-register data, here.\n(data names are defined by what you wire into the bundle function)"
        n80 = Bundle("Core"=w235, "Your Boolean data"=w237, "Your string data"=w236, "Active Module"=w233) -> (w239:T3)  [unwired: 1 in]
        n81 = call <vilib>:"Add State(s) to Queue__JKI_lib_State_Machine.vi"("State(s) in (\"\")"=w241) -> ("States Out"=w240:string)  [unwired: 14 in]
      }
      frame "Data: Cleanup" {
        # "Cleanup any data and references, here.\n(this is called automatically, by the Macro: Exit)"
        n82 = Unbundle By Name(w243) -> ("Core.Current VI Reference"=w246:refnum<vi>)
        n83 = Close Reference(reference=w246, error in (no error)=w245) -> (error out=w244:errorcluster)
        n84 = call <vilib>:"Add State(s) to Queue__JKI_lib_State_Machine.vi"("State(s) in (\"\")"=w248) -> ("States Out"=w247:string)  [unwired: 14 in]
      }
      frame "---------- Events ----------" {
        # "Do not put any code in this frame.\n(It is a separator no-op. You can make a copy of this frame to create a new UI frame)"
        n85 = call <vilib>:"Add State(s) to Queue__JKI_lib_State_Machine.vi"("State(s) in (\"\")"=w253) -> ("States Out"=w252:string)  [unwired: 14 in]
      }
      frame "Events: Register" {
        # "Register message event to break Waiting in Event structure."
        n86 = call "JKISM++ Get New State Notifier Event.vi"("Name(\"\" to use uuid) in"=w256) -> ("Error out"=w254:errorcluster, "New State Notifier Event"=w255:refnum<user-event>)  [unwired: 9 in]
        n87 = register-events(w255) -> (reference out=w257:refnum<event-registration>)  [unwired: 2 in, 1 out]
      }
      frame "Events: Unregister" {
        n88 = Unregister For Events(event registration refnum=w260, error in=w264) -> (error out=w261:errorcluster)
      }
      frame "---------- UI ----------" {
        # "Do not put any code in this frame.\n(It is a separator no-op. You can make a copy of this frame to create a new UI frame)"
        n89 = call <vilib>:"Add State(s) to Queue__JKI_lib_State_Machine.vi"("State(s) in (\"\")"=w269) -> ("States Out"=w268:string)  [unwired: 14 in]
      }
      frame "UI: Initialize" {
        # "Initialize the User Interface, here.\n(this is called automatically, by the Macro: Init)"
        n90 = Unbundle By Name(w271) -> ("Active Module"=w270:string)
        n91 = local write "Target Module"(w270) -> ()
        n92 = call <vilib>:"Add State(s) to Queue__JKI_lib_State_Machine.vi"("State(s) in (\"\")"=w275) -> ("States Out"=w274:string)  [unwired: 14 in]
      }
      frame "UI: Cursor Set" {
        # "Argument"
        # "Set and Unset Cursor Busy.\n(Usage: \"UI: Cursor Set >> Busy|Idle\")"
        n93 = case shown="\"Idle\", Default" w277 {
          tunnel: w279 -> [w284 w286]
          tunnel: [w283 w285] -> w278
          frame "Idle", Default {
            n94 = call <vilib>:"Unset Busy.vi"("error in (no error)"=w284) -> ("error out"=w283:errorcluster)  [unwired: 10 in]
          }
          frame "Busy" {
            n95 = call <vilib>:"Set Busy.vi"("error in (no error)"=w286) -> ("error out"=w285:errorcluster)  [unwired: 9 in, 1 out]
          }
        }
        n96 = call <vilib>:"Add State(s) to Queue__JKI_lib_State_Machine.vi"("State(s) in (\"\")"=w282) -> ("States Out"=w281:string)  [unwired: 14 in]
      }
      frame "UI: Front Panel State" {
        # "Argument"
        # "Set Front Panel Open or Closed\n(Usage: \"UI: Front Panel State >> Open|Close\")"
        n97 = Unbundle By Name(w290) -> ("Core.Current VI Reference"=w289:refnum<vi>)
        n98 = call <vilib>:"Add State(s) to Queue__JKI_lib_State_Machine.vi"("State(s) in (\"\")"=w294) -> ("States Out"=w293:string)  [unwired: 14 in]
        n99 = case shown="\"Minimize\", \"Minimized\"" w288 {
          tunnel: w292 -> [w300 w315 w326 w339 w352]
          tunnel: [w302 w316 w328 w341 w354] -> w291
          tunnel: w289 -> [w301 w313 w327 w340 w353]
          frame "Open", "Standard", Default {
            w295 = T1."Standard" ("State")
            n100 = property class="VI"(reference=w301, error in=w300) -> (reference out=w298:refnum<vi>, error out=w299:errorcluster, "FP.State"=w297:T1)
            n101 = Not Equal?(x=w297, y=w295) -> (x != y?=w296:bool)
            n102 = case shown="True" w296 {
              tunnel: [w306 w308] -> w302
              tunnel: w299 -> [w305 w308]
              tunnel: w298 -> [w304 _]
              tunnel: w295 -> [w303 _]
              frame True {
                n103 = invoke class="VI" method="FP.Open"(reference=w304, error in=w305, "Activate"=TRUE, "State"=w303) -> (error out=w306:errorcluster)  [unwired: 1 in, 4 out]
              }
              frame False {
              }
            }
          }
          frame "Close", "Closed" {
            n104 = property class="VI"(reference=w313, error in=w315) -> (reference out=w312:refnum<vi>, error out=w314:errorcluster, "FP.State"=w310:T1)
            n105 = Not Equal?(x=w310, y=T1."Closed" ("Front Panel Window:State")) -> (x != y?=w309:bool)
            n106 = case shown="True" w309 {
              tunnel: [w317 w320] -> w316
              tunnel: w314 -> [w317 w319]
              tunnel: w312 -> [_ w318]
              frame False {
              }
              frame True {
                n107 = invoke class="VI" method="FP.Close"(reference=w318, error in=w319) -> (error out=w320:errorcluster)  [unwired: 1 in, 2 out]
              }
            }
          }
          frame "Hidden", "Hide" {
            w321 = T1."Hidden" ("State")
            n108 = property class="VI"(reference=w327, error in=w326) -> (reference out=w324:refnum<vi>, error out=w325:errorcluster, "FP.State"=w323:T1)
            n109 = Not Equal?(x=w323, y=w321) -> (x != y?=w322:bool)
            n110 = case shown="True" w322 {
              tunnel: [w332 w333] -> w328
              tunnel: w325 -> [w331 w333]
              tunnel: w324 -> [w330 _]
              tunnel: w321 -> [w329 _]
              frame True {
                n111 = invoke class="VI" method="FP.Open"(reference=w330, error in=w331, "State"=w329) -> (error out=w332:errorcluster)  [unwired: 2 in, 4 out]
              }
              frame False {
              }
            }
          }
          frame "Minimize", "Minimized" {
            w334 = T1."Minimized" ("State")
            n112 = property class="VI"(reference=w340, error in=w339) -> (reference out=w337:refnum<vi>, error out=w338:errorcluster, "FP.State"=w336:T1)
            n113 = Not Equal?(x=w336, y=w334) -> (x != y?=w335:bool)
            n114 = case shown="True" w335 {
              tunnel: [w345 w346] -> w341
              tunnel: w338 -> [w344 w346]
              tunnel: w337 -> [w343 _]
              tunnel: w334 -> [w342 _]
              frame True {
                n115 = invoke class="VI" method="FP.Open"(reference=w343, error in=w344, "State"=w342) -> (error out=w345:errorcluster)  [unwired: 2 in, 4 out]
              }
              frame False {
              }
            }
          }
          frame "Maximize", "Maximized" {
            w347 = T1."Maximized" ("State")
            n116 = property class="VI"(reference=w353, error in=w352) -> (reference out=w350:refnum<vi>, error out=w351:errorcluster, "FP.State"=w349:T1)
            n117 = Not Equal?(x=w349, y=w347) -> (x != y?=w348:bool)
            n118 = case shown="True" w348 {
              tunnel: [w358 w359] -> w354
              tunnel: w351 -> [w357 w359]
              tunnel: w350 -> [w356 _]
              tunnel: w347 -> [w355 _]
              frame True {
                n119 = invoke class="VI" method="FP.Open"(reference=w356, error in=w357, "State"=w355) -> (error out=w358:errorcluster)  [unwired: 2 in, 4 out]
              }
              frame False {
              }
            }
          }
        }
      }
      frame "---------- Macro ----------" {
        # "Do not put any code in this frame.\n(It is a separator no-op. You can make a copy of this frame to create a new Macro frame)"
        n120 = call <vilib>:"Add State(s) to Queue__JKI_lib_State_Machine.vi"("State(s) in (\"\")"=w364) -> ("States Out"=w363:string)  [unwired: 14 in]
      }
      frame "Macro: Initialize" {
        w366 = "Data: Initialize\nInitialize Core Data\nEvents: Register\nUI: Initialize\nUI: Front Panel State >> Open\nMacro: Switch Active Module"  # Data: Initialize Initialize Core Data Events: Register UI: Initialize UI: Front Panel State >> Open Macro: Switch Active Module
        # "Initialization Macro\n(This is called once, when the VI starts)"
        n121 = call <vilib>:"Add State(s) to Queue__JKI_lib_State_Machine.vi"("State(s) in Front (\"\")"=w366, "State(s) in (\"\")"=w370) -> ("States Out"=w369:string)  [unwired: 13 in]
      }
      frame "Macro: Switch Active Module" {
        n122 = Unbundle By Name(w373) -> ("Active Module"=w372:string)
        n123 = call-poly "Build Message with Arguments++.vi"("State with Arguments"="API: Get Level" ("State(s) in Front (\"\")"), "Target Module (\"\")"=w372) -> ("State with Arguments"=w371:string)  [unwired: 13 in]
        n124 = call <vilib>:"Add State(s) to Queue__JKI_lib_State_Machine.vi"("State(s) in Front (\"\")"=w371, "State(s) in (\"\")"=w375) -> ("States Out"=w376:string)  [unwired: 13 in]
      }
      frame "Macro: Exit" {
        # "Exit Macro\n(This is called once, when the VI exits)"
        n125 = Unbundle By Name(w386) -> ("Core.Close Panel on Exit?"=w385:bool)
        n126 = Select(t="UI: Front Panel State >> Close", s=w385, f="") -> (s? t:f=w382:string)
        n127 = call <vilib>:"Add State(s) to Queue__JKI_lib_State_Machine.vi"("State(s) in (\"\")"=w382, "State(s) at Back (\"\")"="Data: Cleanup\nEvents: Unregister\nExit") -> ("States Out"=w380:string)  [unwired: 13 in]
        n128 = call <vilib>:"Add State(s) to Queue__JKI_lib_State_Machine.vi"("State(s) in Front (\"\")"=w380, "State(s) in (\"\")"=w389) -> ("States Out"=w388:string)  [unwired: 13 in]
      }
      frame "------- Action -------" {
      }
      frame "Action: Status Chanage Handler" {
      }
    }
  }
  n129 = call "JKISM-Reuse Module.vi"("Name(\"\" to use uuid)"="SubModule0" ("Name(\"\" to use uuid)")) -> ()  [unwired: 11 in]
  n130 = call "JKISM-Reuse Module.vi"("Name(\"\" to use uuid)"="SubModule1" ("Name(\"\" to use uuid)")) -> ()  [unwired: 11 in]
